vi "GetReason.vi"(10 "condition met":bool, 11 "triggered conditions":T2[](array[typedef])=[{"Condition"={"Source"="", "Type"="", "Operator"="", "CompareTo"="", "DwellSeconds"=0.0}, "LatchValue"="", "LatchTime"=timestamp(0 s since 1904-01-01)}, {"Condition"={"Source"="", "Type"="", "Operator"="", "CompareTo"="", "DwellSeconds"=0.0}, "LatchValue"="", "LatchTime"=timestamp(0 s since 1904-01-01)}]) -> (2 "reason":T1)   [LabVIEW 2017, in "Trigger.lvlib"]
uses:
  <vilib>/addons/InsightCM/Devices/Shared/Common/Trigger/Trigger.lvlib
  <vilib>/addons/InsightCM/Devices/Shared/Common/Trigger/controls/TriggerCondition.ctl
  <vilib>/addons/InsightCM/MessageBus/Base/controls/Condition.ctl
  <vilib>/addons/InsightCM/Devices/Shared/Common/DataEventCreator/controls/Reason.ctl
  <vilib>/addons/InsightCM/Devices/Shared/Common/DataEventCreator/DataEventCreator.lvlib
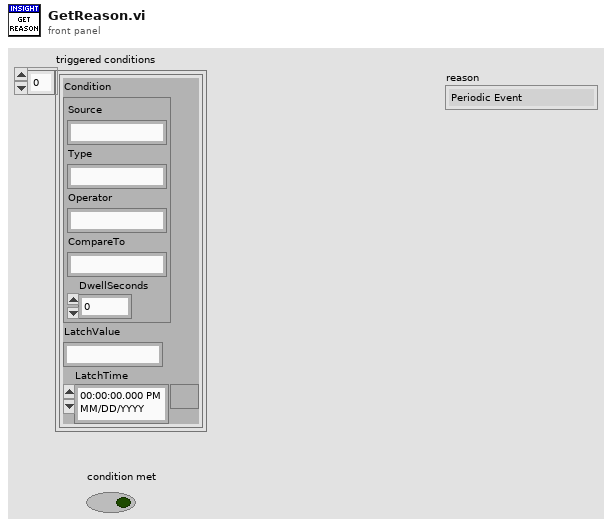
[diagram p1: front panel]
types:
  T1 = typedef "DataEventCreator.lvlib/Reason.ctl" = enum16{"Periodic Event", "Delta EU Event", "Trend Event", "Alarm Event", "User Event", "Enter Operating State", "Exit Operating State", "Multiple Events", "Other"}
  T2 = typedef "Trigger.lvlib/TriggerCondition.ctl" = cluster{"Condition":T3, "LatchValue":string, "LatchTime":timestamp}
  T3 = typedef "Condition.ctl" = cluster{"Source":string, "Type":string, "Operator":string, "CompareTo":string, "DwellSeconds":dbl}
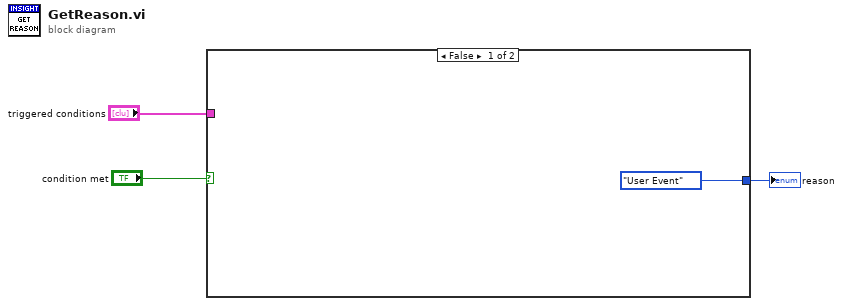
[diagram p0: block diagram]
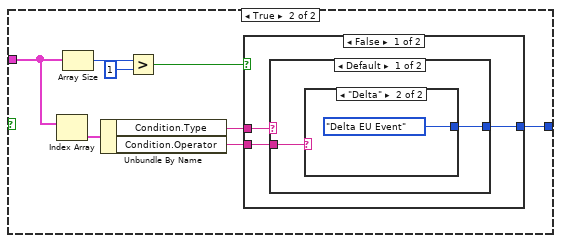
[diagram p2: hidden frame]
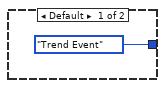
[diagram p3: hidden frame]
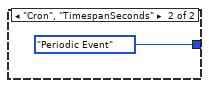
[diagram p4: hidden frame]
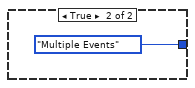
[diagram p5: hidden frame]
diagram:
  n1 = case shown="False" "condition met" {
    tunnel: "triggered conditions" -> [_ w10]
    tunnel: [Reason."User Event" ("Reason") w9] -> w1
    frame False {
    }
    frame True {
      n2 = Index Array(array=w10) -> (element=w8:T2)  [unwired: 1 in]
      n3 = Array Size(array=w10) -> (size(s)=w12:i32)
      n4 = Unbundle By Name(w8) -> ("Condition.Type"=w7:string, "Condition.Operator"=w6:string)
      n5 = Greater?(x=w12, y=1) -> (0:w5:bool)
      n6 = case shown="False" w5 {
        tunnel: [w13 Reason."Multiple Events" ("Reason")] -> w9
        tunnel: w7 -> [w15 _]
        tunnel: w6 -> [w14 _]
        frame False {
          n7 = case shown="Default" w15 {
            tunnel: [w17 Reason."Periodic Event" ("Reason")] -> w13
            tunnel: w14 -> [w16 _]
            frame Default {
              n8 = case shown="\"Delta\"" w16 {
                tunnel: [Reason."Trend Event" ("Reason") Reason."Delta EU Event" ("Reason")] -> w17
                frame Default {
                }
                frame "Delta" {
                }
              }
            }
            frame "Cron", "TimespanSeconds" {
            }
          }
        }
        frame True {
        }
      }
    }
  }
  "reason" <- w1
